vi "confirm time format.vi"(0 "Enable":bool=TRUE, 1 "String timestamp":string, 5 "error in (no error)":errorcluster) -> (14 "Use UTC":bool caption="Cancel", 19 "error out":errorcluster)   [LabVIEW 2012]
doc: "Displays a standard dialog box that prompts users to enter information, such as a user name and password.\n--------------------\n\nThis Express VI is configured as follows:\n\nMessage to Display to the User:Is the time format for this dataset UTC?\nThe inputs are:"
panel:
  out "UTC":bool
  in  "Switch formats":bool
  out "time stamp":timestamp
  out "String":string="Is the time format for this dataset UTC?"
  in  "UTC":bool caption="Cancel"
  in  "Mountain Time":bool caption="OK2"
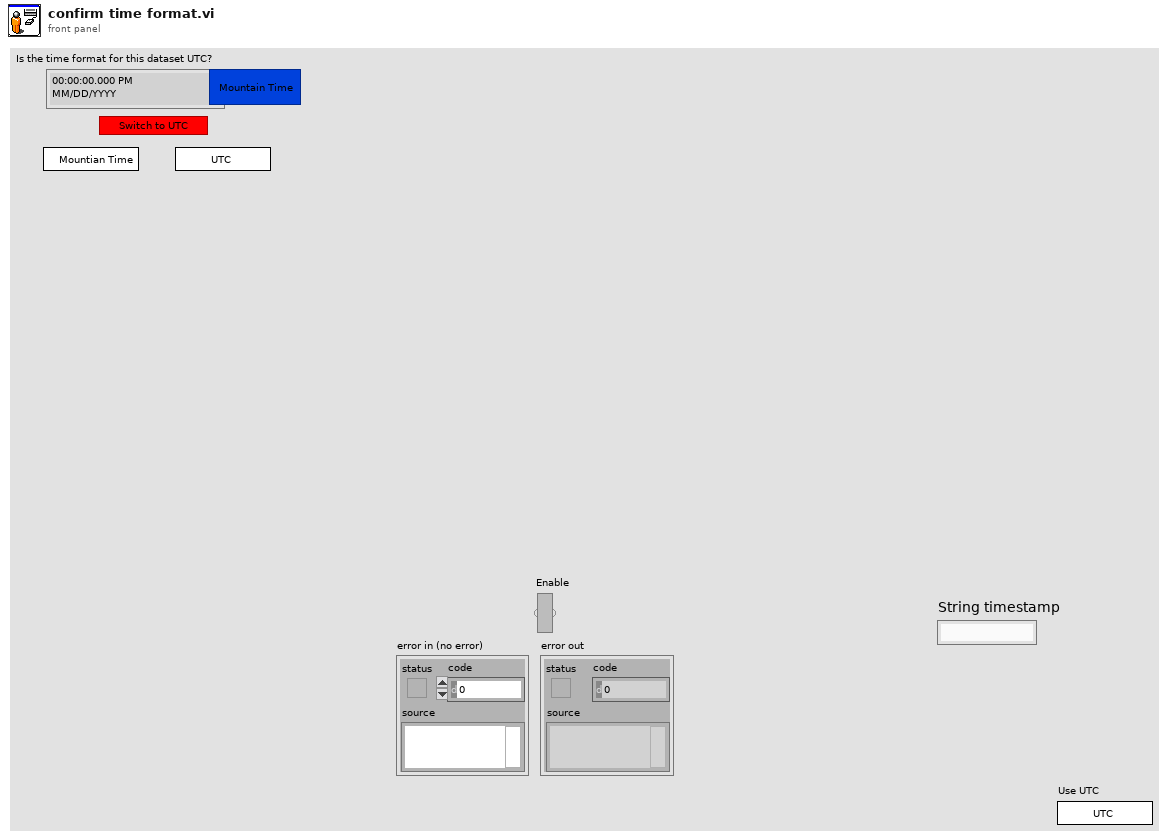
[diagram p1: front panel]
types:
  T1 = cluster{"Input Name":string, "Input Data Type":i32}[]
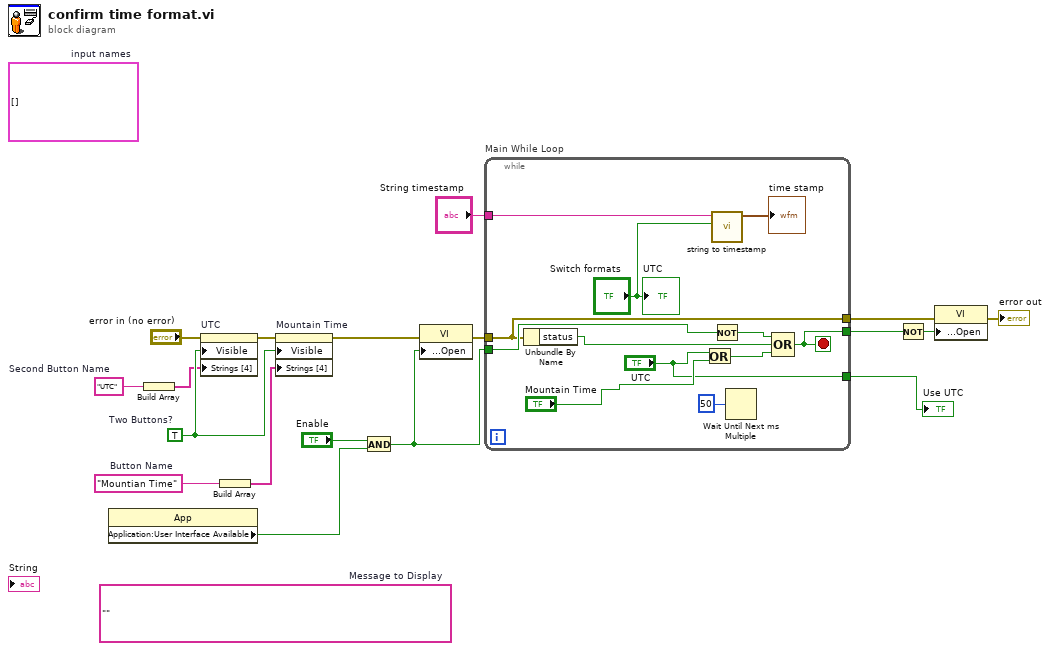
[diagram p0: block diagram]
diagram:
  (unwired) T1 []  # input names
  w13 = "UTC"  # Second Button Name
  w11 = "Mountian Time"  # Button Name
  (unwired) ""  # Message to Display
  w18 = TRUE  # Two Buttons?
  n1 = property class="App"() -> ("Application:User Interface Available"=w4:bool)  [unwired: 2 in, 2 out]
  n2 = Build Array(w13) -> (w14:string[])
  n3 = property on="UTC" class="Bool"(error in="error in (no error)", "Visible"=w18, "Strings [4]"=w14) -> (error out=w17:errorcluster)  [unwired: 1 in, 1 out]
  n4 = Build Array(w11) -> (w12:string[])
  n5 = property on="Mountain Time" class="Bool"(error in=w17, "Visible"=w18, "Strings [4]"=w12) -> (error out=w2:errorcluster)  [unwired: 1 in, 1 out]
  n6 = And(x="Enable", y=w4) -> (x .and. y?=w5:bool)
  n7 = property class="VI"(error in=w2, "Front Panel Window:Open"=w5) -> (error out=w10:errorcluster)  [unwired: 1 in, 1 out]
  n8 = while "Main While Loop" {
    tunnel: w5 -> [w29]
    tunnel: [w27] -> w15
    tunnel: w10 -> [w26]
    tunnel: [w26] -> w8
    tunnel: "String timestamp" -> [w23]
    tunnel: ["UTC"] -> w1
    stop <- w27 stop-if-true
    n9 = Unbundle By Name(w26) -> ("status"=w24:bool)
    n10 = Or(x="UTC", y="Mountain Time") -> (x .or. y?=w25:bool)
    n11 = call "string to timestamp.vi"("is UTC (F)"="Switch formats", "string"=w23) -> ("time stamp"=→"time stamp":timestamp)  [unwired: 9 in]
    n12 = Not(x=w29) -> (.not. x?=w28:bool)
    n13 = Wait Until Next ms Multiple(millisecond multiple=u32 50) -> ()  [unwired: 1 out]
    n14 = Compound Arithmetic op=OR(w28, w24, w25) -> (w27:bool)
    "UTC" <- "Switch formats"
  }
  "Use UTC" <- w1
  n15 = Not(x=w15) -> (.not. x?=w16:bool)
  n16 = property class="VI"(error in=w8, "Front Panel Window:Open"=w16) -> (error out=→"error out":errorcluster)  [unwired: 1 in, 1 out]
